vi "Hightlight Color Write.vi"(4 "error in (no error)":errorcluster, 5 "Value":T1, 6 "Container State":T3, 7 "Display State In":T2={"Persistent"={"Elements"=[], "PicElements"=[], "Limits"=[], "Selection"=[], "Selection Color"=0, "Highlight"=[], "Highlight Val"=0, "Highlight Color"={"Back"=0, "Edge"=0}, "Font"={"Details"={"Font Name:"="Lucida Sans", "Size"=24, "Strikeout?"=FALSE, "Italic?"=FALSE, "Underline?"=FALSE, "Outline?"=FALSE, "Shadow?"=FALSE, "Bold?"=TRUE}, "Color"=7697781}, "Bakground Color"=0}, "List Ref"=refnum, "nbVisible"=0, "FirstIdx"=0, "More.Width"=0}) -> (0 "error out":errorcluster, 3 "Display State Out":T2={"Persistent"={"Elements"=[], "PicElements"=[], "Limits"=[], "Selection"=[], "Selection Color"=0, "Highlight"=[], "Highlight Val"=0, "Highlight Color"={"Back"=0, "Edge"=0}, "Font"={"Details"={"Font Name:"="Lucida Sans", "Size"=24, "Strikeout?"=FALSE, "Italic?"=FALSE, "Underline?"=FALSE, "Outline?"=FALSE, "Shadow?"=FALSE, "Bold?"=TRUE}, "Color"=7697781}, "Bakground Color"=0}, "List Ref"=refnum, "nbVisible"=0, "FirstIdx"=0, "More.Width"=0})   [LabVIEW 2016, in "Horizontal MenuList.xctl"]
uses:
  Horizontal MenuList.xctl
  <vilib>/_xctls/Container State.ctl
  Horizontal MenuList_State.ctl
  _SubVIs/Highlight Colors.ctl
  <vilib>/_xctls/XControlSupport.lvlib
panel:
  # "Replace the Value Control below with a Control of desired type.\nDo not remove this Control or the others from the connector pane.\nDo not change the connector pane pattern.\nThe Value control should always be the third terminal from top on the input side in the connector pane."
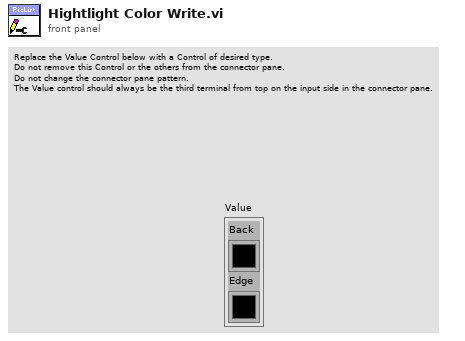
[diagram p1: front panel]
types:
  T1 = typedef "Horizontal MenuList.xctl/Highlight Colors.ctl" = cluster{"Back":u32, "Edge":u32}
  T2 = typedef "Horizontal MenuList.xctl/Horizontal MenuList_State.ctl" = cluster{"Persistent":cluster{"Elements":string[], "PicElements":picture[], "Limits":i32[], "Selection":picture[], "Selection Color":u32, "Highlight":picture[], "Highlight Val":i32, "Highlight Color":T1, "Font":cluster{"Details":cluster{"Font Name:":string, "Size":i16, "Strikeout?":bool, "Italic?":bool, "Underline?":bool, "Outline?":bool, "Shadow?":bool, "Bold?":bool}, "Color":u32}, "Bakground Color":u32}, "List Ref":refnum<vi>, "nbVisible":u8, "FirstIdx":u8, "More.Width":u8}
  T3 = typedef "XControlSupport.lvlib/Container State.ctl" = cluster{"Indicator?":bool, "Run Mode?":bool, " Refnum":refnum<vi>}
  T4 = typedef "LVBoundsTypeDef.ctl" = cluster{"Width":u32, "Height":u32}
  T5 = cluster{"left":i16, "top":i16, "right":i16, "bottom":i16}
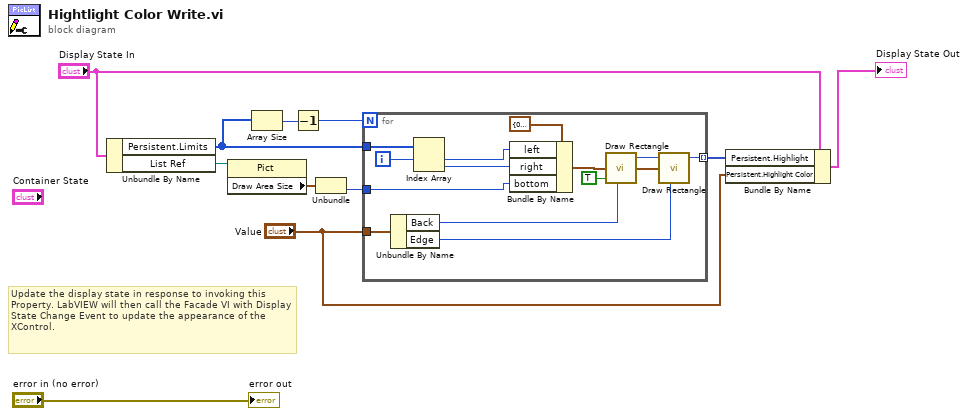
[diagram p0: block diagram]
diagram:
  # "Update the display state in response to invoking this Property. LabVIEW will then call the Facade VI with Display State Change Event to update the appearance of the XControl."
  n1 = Unbundle By Name("Display State In") -> ("Persistent.Limits"=w8:i32[], "List Ref"=w7:refnum<vi>)
  n2 = property class="Pict"(reference=w7) -> ("Draw Area Size"=w2:T4)  [unwired: 1 in, 2 out]
  n3 = Array Size(array=w8) -> (size(s)=w10:i32)
  n4 = Decrement(x=w10) -> (x-1=w9:i32)
  n5 = Unbundle(w2) -> ("Height"=w1:u32)  [unwired: 1 out]
  n6 = for {
    N: w9 -> [_]
    tunnel: w8 -> [w18]
    tunnel: "Value" -> [w22]
    tunnel: [w19] -> w4 mode=indexing
    tunnel: w1 -> [w12]
    i -> [w17]
    n7 = Unbundle By Name(w22) -> ("Back"=w21:u32, "Edge"=w20:u32)
    n8 = Index Array(array=w18, index #1=w17) -> (element #1=w14:i32, element #2=w13:i32)  [unwired: 1 in]
    n9 = Bundle By Name(cluster=T5 {"left"=0, "top"=0, "right"=0, "bottom"=0} ("rect"), "left"=w14, "right"=w13, "bottom"=w12) -> (w15:T5)
    n10 = call <vilib>:"Draw Rectangle.vi"("rect"=w15, "fill?(F)"=TRUE, "color(black)"=w21) -> ("new picture"=w23:picture)  [unwired: 6 in]
    n11 = call <vilib>:"Draw Rectangle.vi"("picture"=w23, "rect"=w15, "color(black)"=w20) -> ("new picture"=w19:picture)  [unwired: 6 in]
  }
  n12 = Bundle By Name(cluster="Display State In", "Persistent.Highlight"=w4, "Persistent.Highlight Color"="Value") -> (→"Display State Out":T2)
  "error out" <- "error in (no error)"
